vi "RF Switch tool.vi"(4 "error in":errorcluster, 5 "Index":i8 min=0 max=24, 6 "array input":bool[][](array[boolean])=array80x96[7680 elements], 7 "DAQ Device":enum16{"Dev1", "Dev2", "Dev3"}(ring)) -> (0 "Error out":errorcluster={"status"=TRUE, "code"=-201003, "source"="DAQmx Create Channel (DO-Digital Output).vi:1<append>\n<B>指定的设备: </B>Dev1\n\n<B>任务名称: </B>_unnamedTask<0>"})   [LabVIEW 2011]
uses:
  <vilib>/Utility/error.llb/DialogType.ctl
  <vilib>/Utility/file.llb/Read From Spreadsheet File (I64).vi
  <vilib>/Utility/file.llb/Write To Spreadsheet File (I64).vi
panel:
  in  "Index":i32[](array[numeric])=[1, 2, 3, 4, 5, 6, 7, 8, 9, 10, 11, 12, 13, 14, 15, 16, 17, 18, 19, 20, 21, 22, 23, 24, 25, 26, 27, 28, 29, 30, 31, 32, 33, 34, 35, 36, 37, 38, 39, 40, 41, 42, 43, 44, 45, 46, 47, 48, 49, 50, 51, 52, 53, 54, 55, 56, 57, 58, 59, 60, 61, 62, 63, 64, 65, 66, 67, 68, 69, 70, 71, 72, 73, 74, 75, 76, 77, 78, 79, 80]
  in  "PCI-6509: P0-P1-P2-P3-P4-P5":dbl[](array[numeric])=[0.0, 1.0, 2.0, 3.0, 4.0, 5.0, 6.0, 7.0, 0.0, 1.0, 2.0, 3.0, 4.0, 5.0, 6.0, 7.0, 0.0, 1.0, 2.0, 3.0, 4.0, 5.0, 6.0, 7.0, 0.0, 1.0, 2.0, 3.0, 4.0, 5.0, 6.0, 7.0, 0.0, 1.0, 2.0, 3.0, 4.0, 5.0, 6.0, 7.0, 0.0, 1.0, 2.0, 3.0, 4.0, 5.0, 6.0, 7.0]
  in  "Switch Matrix":u16(ring) items=["999.dat", "Internal Mini-SAS.dat", "QSFP+ - 副本.dat", "QSFP+.dat", "SFP+.dat"]
  in  "Basic Path":path=path "C:/Users/L025200.LUXSHARE/Desktop/VNA Aotomatic Data Save Tool 20150327/Switch Matrix"
  out "Matrix List":string[](array[string])
  out "Path":path=path "C:/Users/L025200.LUXSHARE/Desktop/VNA Aotomatic Data Save Tool 20150327/Switch Matrix"
  in  "Modify":bool
  in  "Lines 4":tag="Dev3/port0/line0:7, Dev3/port1/line0:7, Dev3/port2/line0:7, Dev3/port3/line0:7, Dev3/port4/line0:7, Dev3/port5/line0:7, Dev3/port6/line0:7, Dev3/port7/line0:7, Dev3/port8/line0:7, Dev3/port9/line0:7, Dev3/port10/line0:7, Dev3/port11/line0:7" caption="Lines"
  in  "Lines 2":tag="Dev2/port0/line0:7, Dev2/port1/line0:7, Dev2/port2/line0:7, Dev2/port3/line0:7, Dev2/port4/line0:7, Dev2/port5/line0:7, Dev2/port6/line0:7, Dev2/port7/line0:7, Dev2/port8/line0:7, Dev2/port9/line0:7, Dev2/port10/line0:7, Dev2/port11/line0:7" caption="Lines"
  in  "Lines":tag="Dev1/port0/line0:7, Dev1/port1/line0:7, Dev1/port2/line0:7, Dev1/port3/line0:7, Dev1/port4/line0:7, Dev1/port5/line0:7, Dev1/port6/line0:7, Dev1/port7/line0:7, Dev1/port8/line0:7, Dev1/port9/line0:7, Dev1/port10/line0:7, Dev1/port11/line0:7"
  # "RF Matrix Control System By NI PCI-6509 DAQmx Card"
  # "20150714"
  # "-------------P0------------"
  # "-------------P1------------"
  # "-------------P2------------"
  # "-------------P3------------"
  # "-------------P4------------"
  # "-------------P5------------"
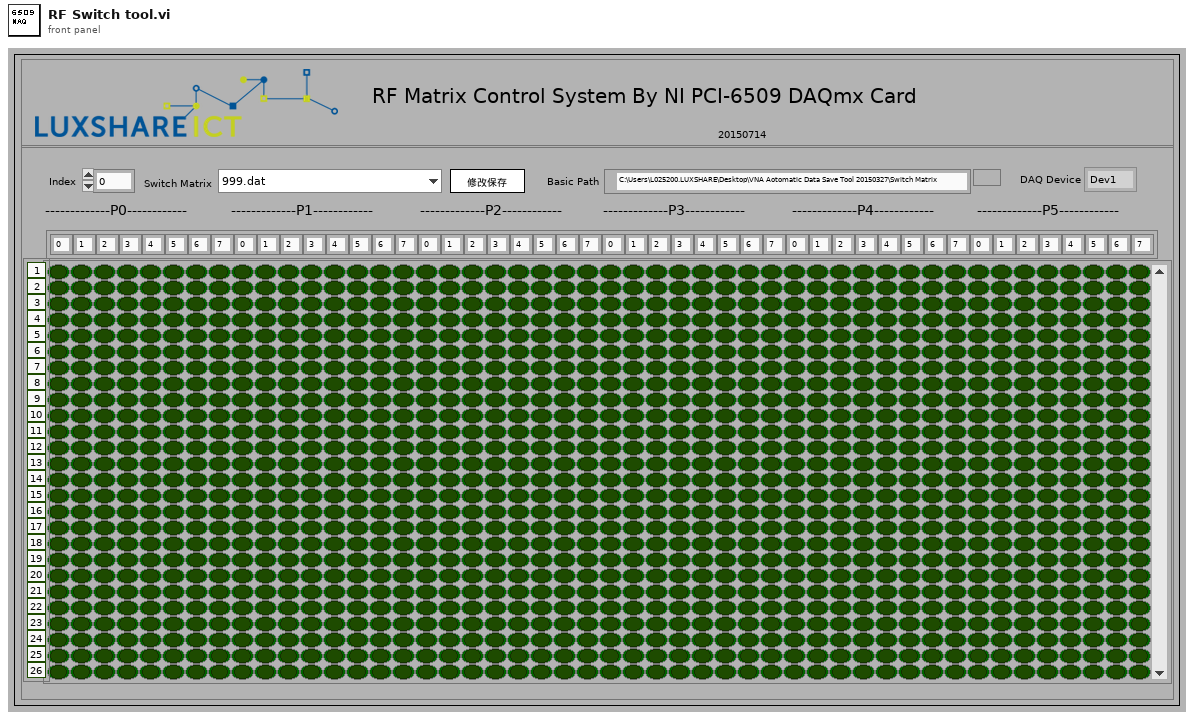
[diagram p1: front panel]
types:
  T1 = typedef "DialogType.ctl" = u16
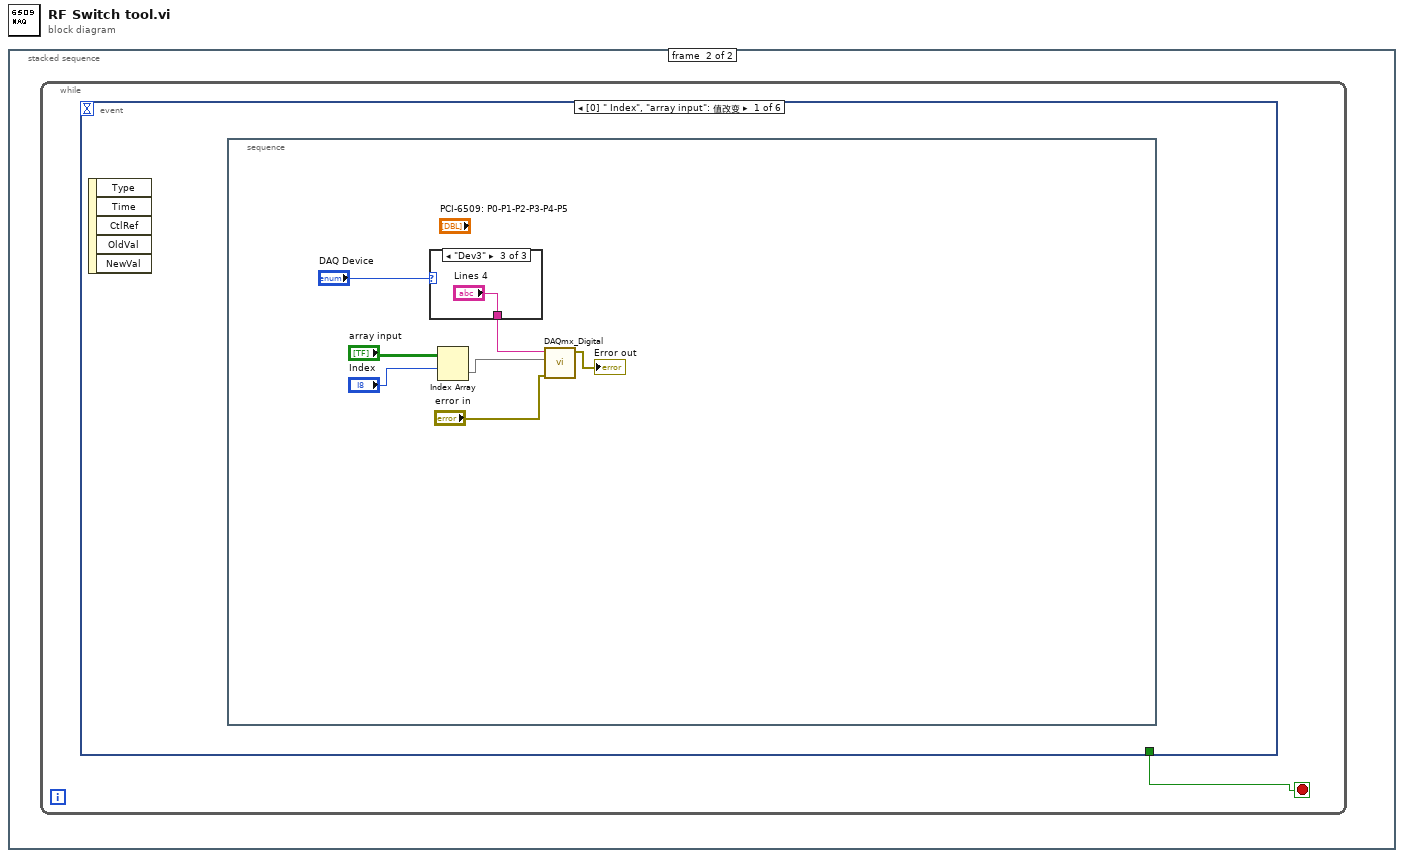
[diagram p0: block diagram]
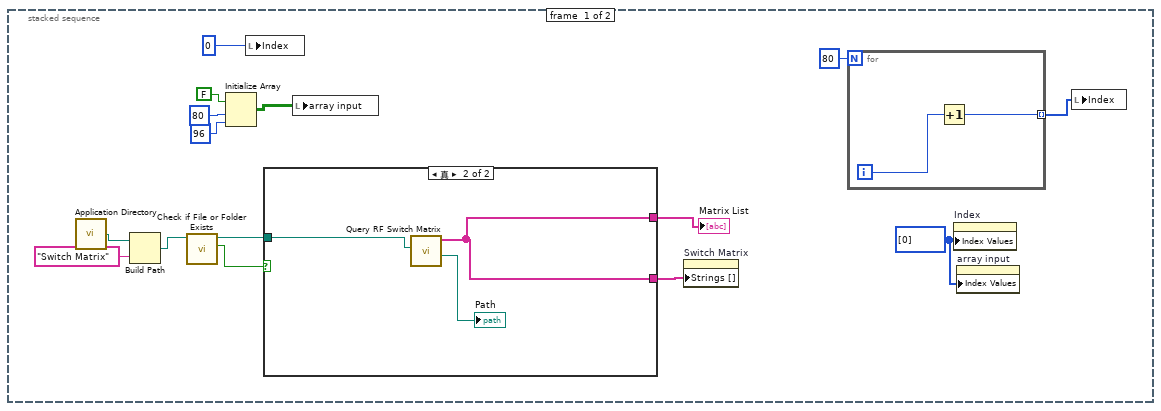
[diagram p2: hidden frame]
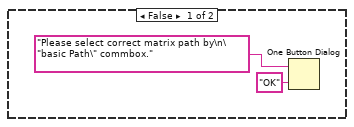
[diagram p3: hidden frame]
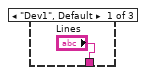
[diagram p4: hidden frame]
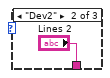
[diagram p5: hidden frame]
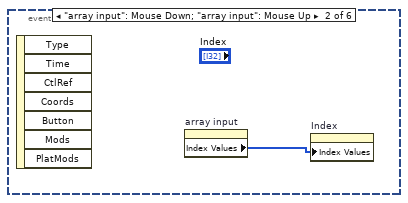
[diagram p6: hidden frame]
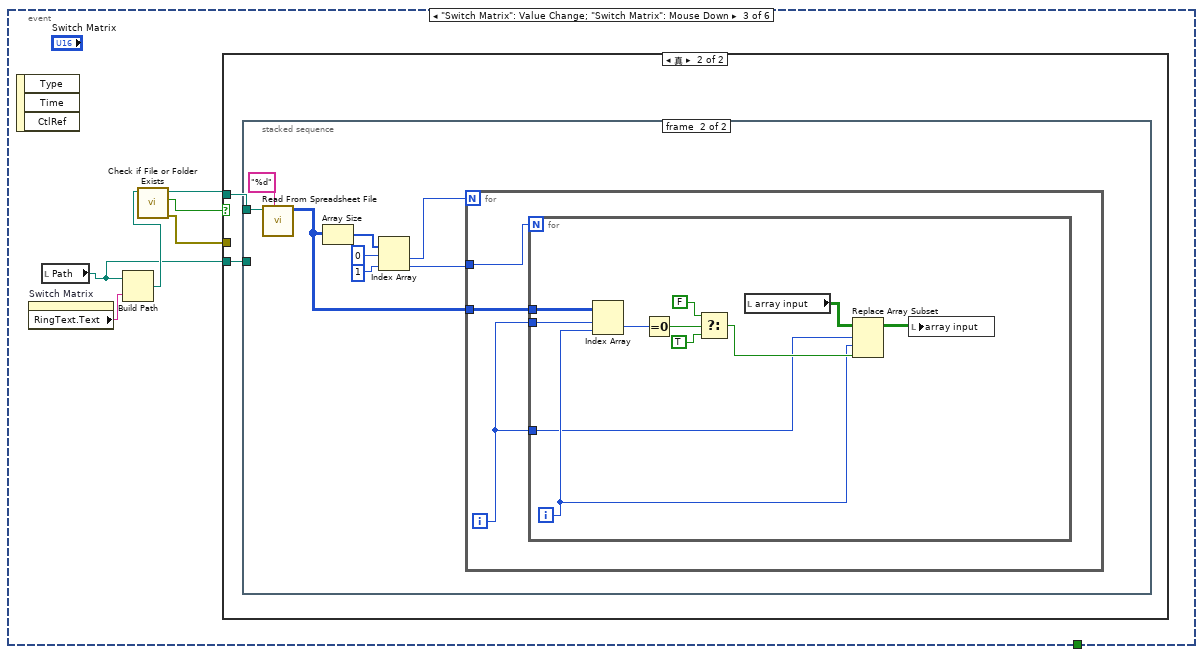
[diagram p7: hidden frame]
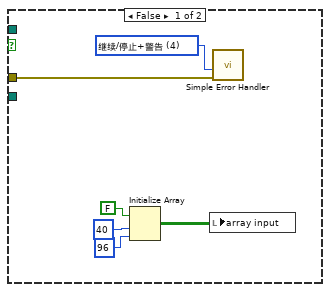
[diagram p8: hidden frame]
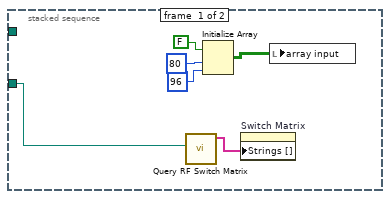
[diagram p9: hidden frame]
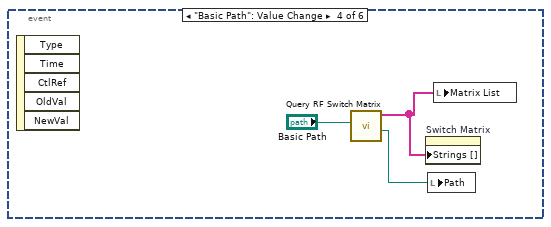
[diagram p10: hidden frame]
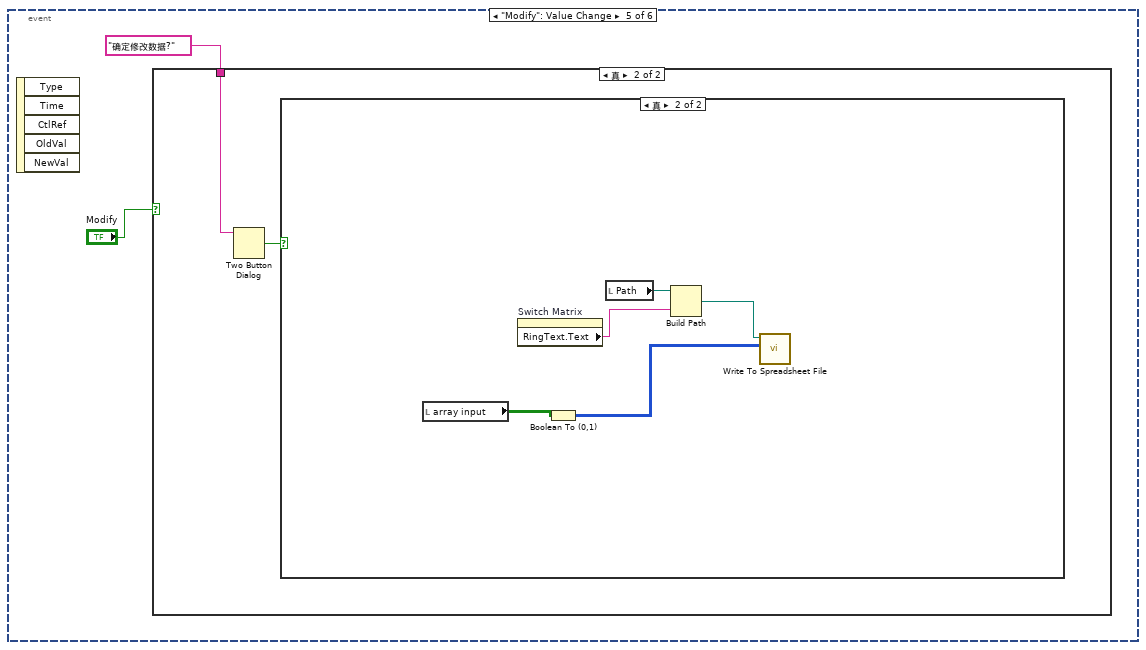
[diagram p11: hidden frame]
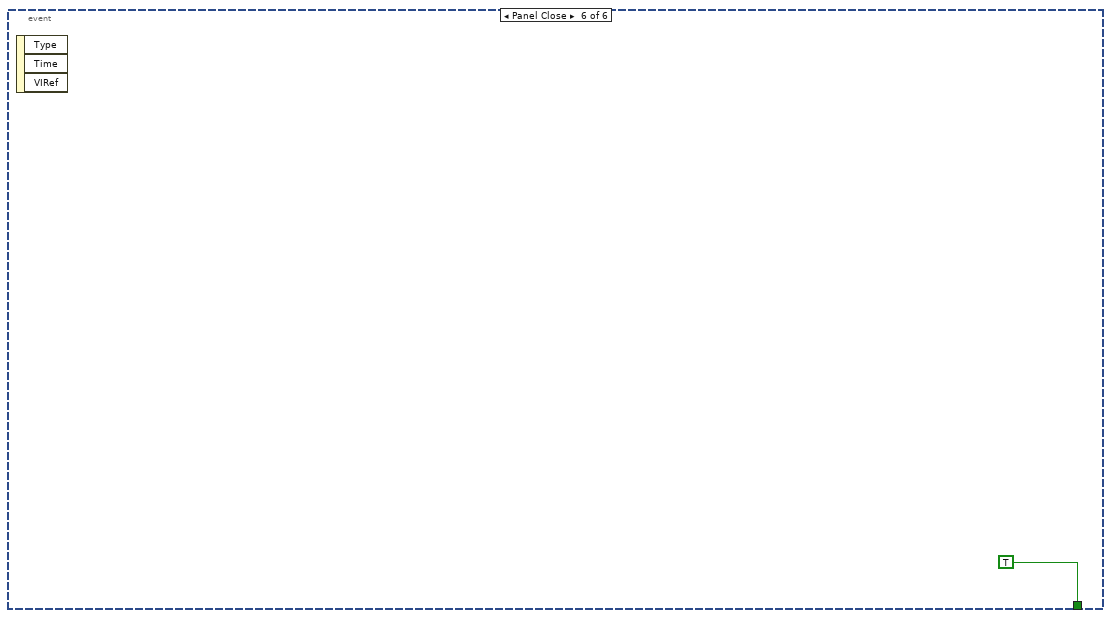
[diagram p14: hidden frame]
diagram:
  n1 = stacked-sequence {
    frame #0 {
      w3 = u32[] [0] ("索引值")
      n2 = call <vilib>:"Application Directory.vi"() -> ("Application Directory"=w10:path)
      n3 = Build Path(base path=w10, name or relative path="Switch Matrix" ("名称或相对路径")) -> (appended path=w8:path)
      n4 = call <vilib>:"Check if File or Folder Exists.vi"("path"=w8) -> ("file or folder exists?"=w7:bool, "dup path"=w6:path)  [unwired: 8 in, 1 out]
      n5 = Initialize Array(FALSE, 80 ("维数大小"), 96 ("维数大小")) -> (w11:bool[][])
      n6 = local write "Index"(i8 0 ("Action Index)")) -> ()
      n7 = case shown="真" w7 {
        tunnel: w6 -> [_ w21]
        tunnel: [_ w20] -> w5
        tunnel: [_ w20] -> w4
        frame False {
          n8 = One Button Dialog(message="Please select correct matrix path by\n\"basic Path\" commbox." ("消息"), button name ("OK")="OK" ("按钮名称（“确定”）")) -> ()  [unwired: 1 out]
        }
        frame True {
          n9 = call "Query RF Switch Matrix.vi"("Basic Path"=w21) -> ("Path"=→"Path":path, "Matrix List"=w20:string[])  [unwired: 9 in]
        }
      }
      "Matrix List" <- w5
      n10 = local write "array input"(w11) -> ()
      n11 = property on="Switch Matrix" class="Ring (严格)"("Strings []"=w4) -> ()  [unwired: 2 in, 2 out]
      n12 = for {
        N: 80 -> [_]
        tunnel: [w16] -> w1 mode=indexing
        i -> [w17]
        n13 = Increment(x=w17) -> (x+1=w16:i32)
      }
      n14 = property on="Index" class="Arr (严格)"("Index Values"=w3) -> ()  [unwired: 2 in, 2 out]
      n15 = property on="array input" class="Arr (严格)"("Index Values"=w3) -> ()  [unwired: 2 in, 2 out]
      n16 = local write "Index"(w1) -> ()
    }
    frame #1 {
      n17 = while {
        stop <- w23 stop-if-true
        n18 = event shown="[0] \" Index\", \"array input\": 值改变" {
          selector: _ -> [_ _ _ _ _ _]
          dyn-events: _ -> [_ _ _ _ _ _]
          timeout: _ -> [_ _ _ _ _ _]
          tunnel: [_ _ _ _ _ TRUE] -> w23
          event "Index", "array input": Value Change {
            n19 = event-data() -> ()  [unwired: 1 in, 5 out]
            n20 = stacked-sequence {
              frame #0 {
                n21 = case shown="\"Dev3\"" "DAQ Device" {
                  tunnel: ["Lines" "Lines 2" "Lines 4"] -> w27
                  frame "Dev1", Default {
                  }
                  frame "Dev2" {
                  }
                  frame "Dev3" {
                  }
                }
                n22 = Index Array(array="array input", index (row)="Index") -> (element=w26:bool[])  [unwired: 1 in]
                n23 = call "DAQmx_Digital.vi"("Error in"="error in", "Data"=w26, "lines"=w27) -> ("Error out"=→"Error out":errorcluster)  [unwired: 8 in]
              }
            }
          }
          event "array input": Mouse Down; "array input": Mouse Up {
            n24 = event-data() -> ()  [unwired: 1 in, 7 out]
            n25 = property on="array input" class="Arr (严格)"() -> ("Index Values"=w34:u32[])  [unwired: 2 in, 2 out]
            n26 = property on="Index" class="Arr (严格)"("Index Values"=w34) -> ()  [unwired: 2 in, 2 out]
          }
          event "Switch Matrix": Value Change; "Switch Matrix": Mouse Down {
            n27 = event-data() -> ()  [unwired: 1 in, 3 out]
            n28 = property on="Switch Matrix" class="Ring (严格)"() -> ("RingText.Text"=w40:string)  [unwired: 2 in, 2 out]
            n29 = local read "Path"() -> (w35:path)
            n30 = Build Path(base path=w35, name or relative path=w40) -> (appended path=w39:path)
            n31 = call <vilib>:"Check if File or Folder Exists.vi"("path"=w39) -> ("error out"=w38:errorcluster, "file or folder exists?"=w37:bool, "dup path"=w36:path)  [unwired: 8 in]
            n32 = case shown="真" w37 {
              tunnel: w38 -> [w46 _]
              tunnel: w36 -> [_ w48]
              tunnel: w35 -> [_ w47]
              frame False {
                w45 = T1 4 items=["无对话框", "确定信息", "继续或停止信息", "确定信息＋警告", "继续/停止+警告"] ("type of dialog (OK msg:1)")
                n33 = Initialize Array(FALSE, 40 ("维数大小"), 96 ("维数大小")) -> (w41:bool[][])
                n34 = local write "array input"(w41) -> ()
                n35 = call <vilib>:"Simple Error Handler.vi"("type of dialog (OK msg:1)"=w45, "error in (no error)"=w46) -> ()  [unwired: 3 in, 5 out]
              }
              frame True {
                n36 = stacked-sequence {
                  tunnel: w48 -> [_ w55]
                  tunnel: w47 -> [w50 _]
                  frame #0 {
                    n37 = call "Query RF Switch Matrix.vi"("Basic Path"=w50) -> ("Matrix List"=w49:string[])  [unwired: 9 in, 1 out]
                    n38 = Initialize Array(FALSE, 80 ("维数大小"), 96 ("维数大小")) -> (w51:bool[][])
                    n39 = property on="Switch Matrix" class="Ring (严格)"("Strings []"=w49) -> ()  [unwired: 2 in, 2 out]
                    n40 = local write "array input"(w51) -> ()
                  }
                  frame #1 {
                    n41 = call-poly <vilib>:"Read From Spreadsheet File.vi"("format (%d)"="%d" ("format (%.3f)"), "file path (dialog if empty)"=w55) -> ("all rows"=w62:i64[][])  [unwired: 5 in, 4 out]
                    n42 = Array Size(array=w62) -> (size(s)=w56:i32[])
                    n43 = Index Array(array=w56, index #1=0 ("索引"), index #2=1 ("索引")) -> (element #1=w59:i32, element #2=w60:i32)
                    n44 = for {
                      N: w59 -> [_]
                      tunnel: w60 -> [w65]
                      tunnel: w62 -> [w64]
                      i -> [w63]
                      n45 = for {
                        N: w65 -> [_]
                        tunnel: w64 -> [w76]
                        tunnel: w63 -> [w75]
                        tunnel: w63 -> [w68]
                        i -> [w69]
                        n46 = Index Array(array=w76, index (row)=w75, index (col)=w69) -> (element=w74:i64)
                        n47 = Equal To 0?(x=w74) -> (x = 0?=w73:bool)
                        n48 = Select(t=FALSE, s=w73, f=TRUE) -> (s? t:f=w70:bool)
                        n49 = local read "array input"() -> (w66:bool[][])
                        n50 = Replace Array Subset(array=w66, new element=w70, index (row)=w68, index (col)=w69) -> (w67:bool[][])
                        n51 = local write "array input"(w67) -> ()
                      }
                    }
                  }
                }
              }
            }
          }
          event "Basic Path": Value Change {
            n52 = event-data() -> ()  [unwired: 1 in, 5 out]
            n53 = call "Query RF Switch Matrix.vi"("Basic Path"="Basic Path") -> ("Path"=w78:path, "Matrix List"=w79:string[])  [unwired: 9 in]
            n54 = property on="Switch Matrix" class="Ring (严格)"("Strings []"=w79) -> ()  [unwired: 2 in, 2 out]
            n55 = local write "Path"(w78) -> ()
            n56 = local write "Matrix List"(w79) -> ()
          }
          event "Modify": Value Change {
            n57 = event-data() -> ()  [unwired: 1 in, 5 out]
            n58 = case shown="真" "Modify" {
              tunnel: "确定修改数据?" ("消息") -> [_ w83]
              frame False {
              }
              frame True {
                n59 = Two Button Dialog(message=w83) -> (T button?=w82:bool)  [unwired: 2 in]
                n60 = case shown="真" w82 {
                  frame False {
                  }
                  frame True {
                    n61 = local read "array input"() -> (w88:bool[][])
                    n62 = property on="Switch Matrix" class="Ring (严格)"() -> ("RingText.Text"=w84:string)  [unwired: 2 in, 2 out]
                    n63 = Boolean To (0,1)(Boolean=w88) -> (0, 1=w87:i16[][])
                    n64 = local read "Path"() -> (w85:path)
                    n65 = Build Path(base path=w85, name or relative path=w84) -> (appended path=w86:path)
                    n66 = call-poly <vilib>:"Write To Spreadsheet File.vi"("2D data"=w87, "file path (dialog if empty)"=w86) -> ()  [unwired: 6 in, 1 out]
                  }
                }
              }
            }
          }
          event Panel Close {
            n67 = event-data() -> ()  [unwired: 1 in, 3 out]
          }
        }
      }
    }
  }
